vi "basic.vi"() -> ()   [LabVIEW 2012]
uses:
  <vilib>/Instr/_visa.llb/VISA Configure Serial Port (Instr).vi
panel:
  in  "stop":bool
  out "read buffer":string
  in  "Com port":refnum<visa-resource-name>
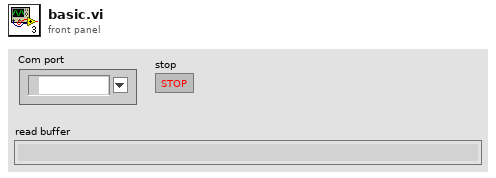
[diagram p1: front panel]
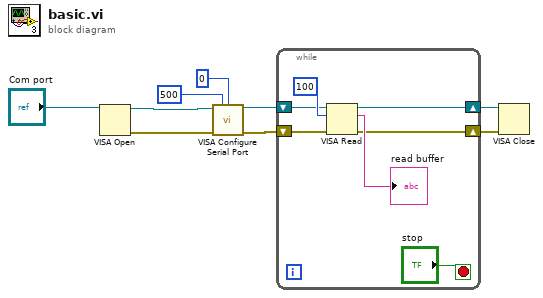
[diagram p0: block diagram]
diagram:
  n1 = VISA Open(VISA resource name="Com port") -> (VISA resource name=w6:refnum<visa-resource-name>, error out=w7:errorcluster)  [unwired: 4 in]
  n2 = call-poly "VISA Configure Serial Port"("VISA resource name"=w6, "timeout (10sec)"=u32 500, "termination char\n(0xA = '\\n' = LF)"=u8 0 ("termination char\n(0xA = '\\n' = LF)"), "error in (no error)"=w7) -> ("VISA resource name out"=w4:refnum<visa-resource-name>, "error out"=w3:errorcluster)  [unwired: 10 in]
  n3 = while {
    shift-right: [w11] -> w1
    shift-left: w3 -> [w13]
    shift-right: [w12] -> w2
    shift-left: w4 -> [w14]
    stop <- "stop" stop-if-true
    n4 = VISA Read(VISA resource name=w14, byte count=u32 100, error in (no error)=w13) -> (VISA resource name out=w12:refnum<visa-resource-name>, read buffer=→"read buffer":string, error out=w11:errorcluster)  [unwired: 1 out]
  }
  n5 = VISA Close(VISA resource name=w2, error in (no error)=w1) -> ()  [unwired: 1 out]
